vi "mqttCmdBuildPayloadInternal.vi"(8 "error in (no error)":errorcluster, 11 "mqttCmdConnect in":refnum<class "ConnectMqttMsg.lvclass">) -> (0 "error out":errorcluster, 2 "payload":u8[](array[numeric]) format="%x", 3 "mqttCmdConnect out":refnum<class "ConnectMqttMsg.lvclass">)   [LabVIEW 2020, in "ConnectMqttMsg.lvclass"]
uses:
  ConnectMqttMsg.lvclass
  ConnectMqttMsg.lvclass/ConnectMqttMsg.ctl
  BaseMqttMsg.lvclass
panel:
  out "willMessage out":u8[](array[numeric])
  out "userInfo out":u8[](array[numeric])
  out "clientID out":u8[](array[numeric])
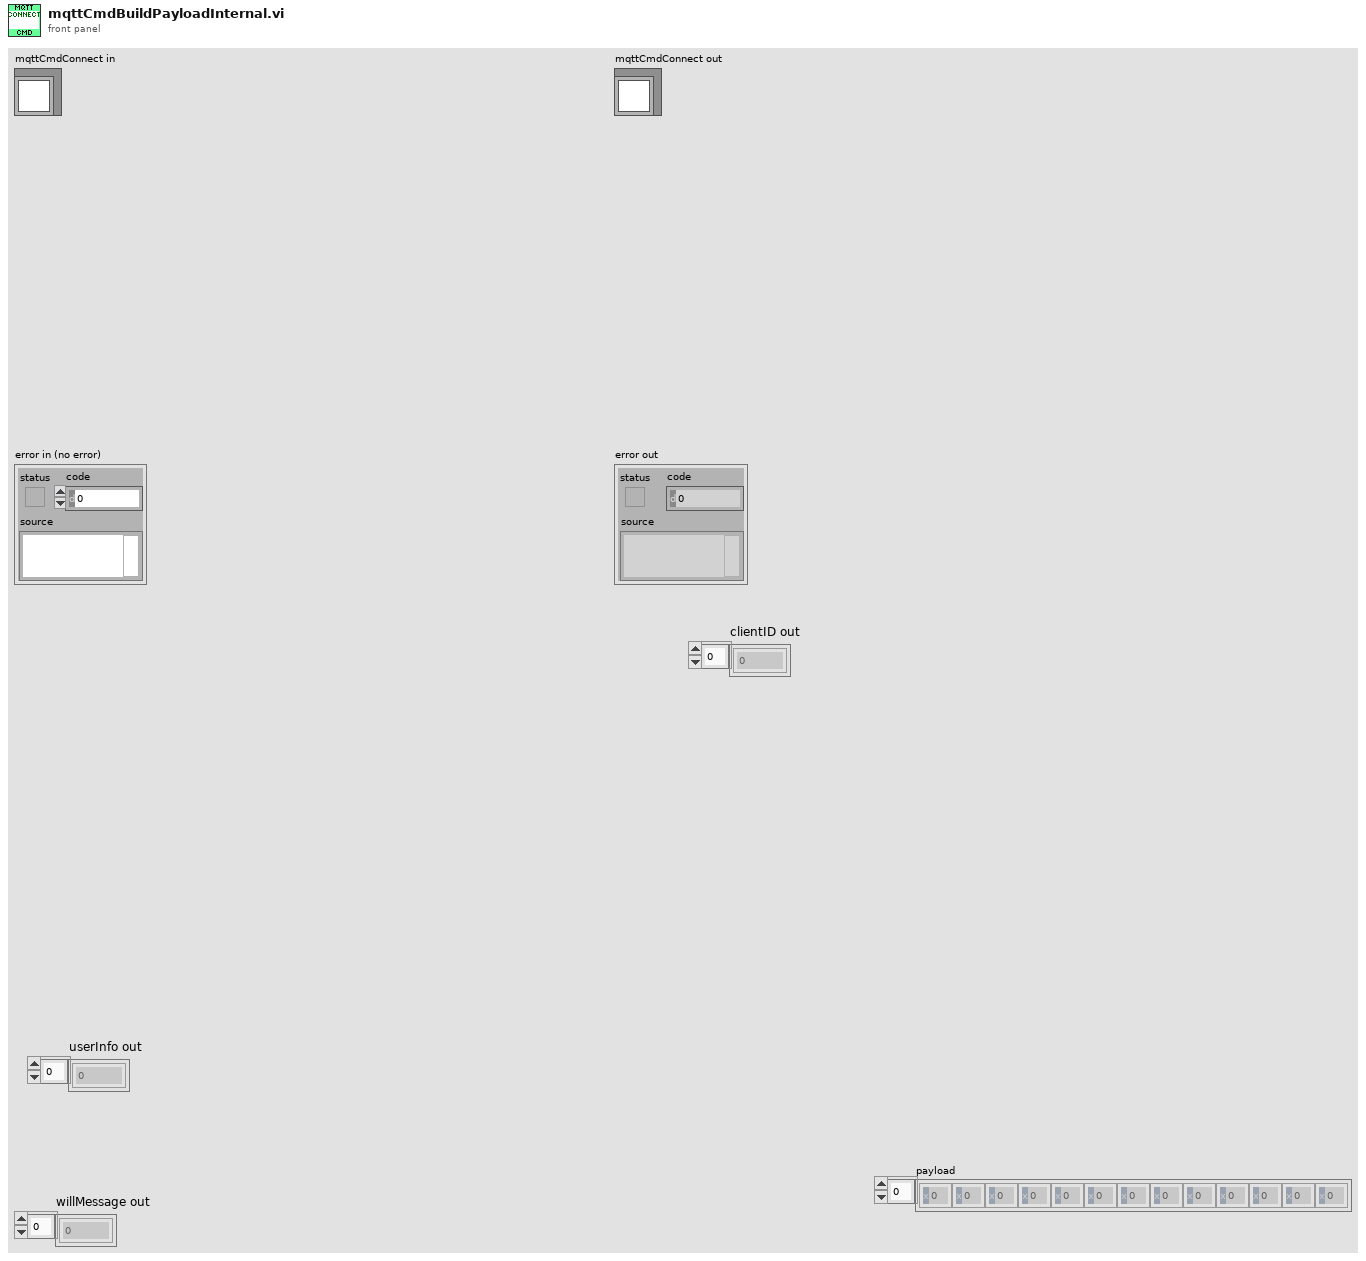
[diagram p1: front panel]
types:
  T1 = typedef "MQTT Client.lvclass/WillDefinition.ctl" = cluster{"Will message":string, "Will Topic":string}
  T2 = typedef "MQTT Client.lvclass/UserCredentials.ctl" = cluster{"User Name":string, "Password":string}
  T3 = typedef "MQTT Client.lvclass/ConnectionFlags.ctl" = cluster{"user name":bool, "password":bool, "will retain":bool, "will flag":bool, "clean session":bool, "reserved":bool, "willQOS":enum8{"At most once", "At least once", "Exactly once", "Reserved"}}
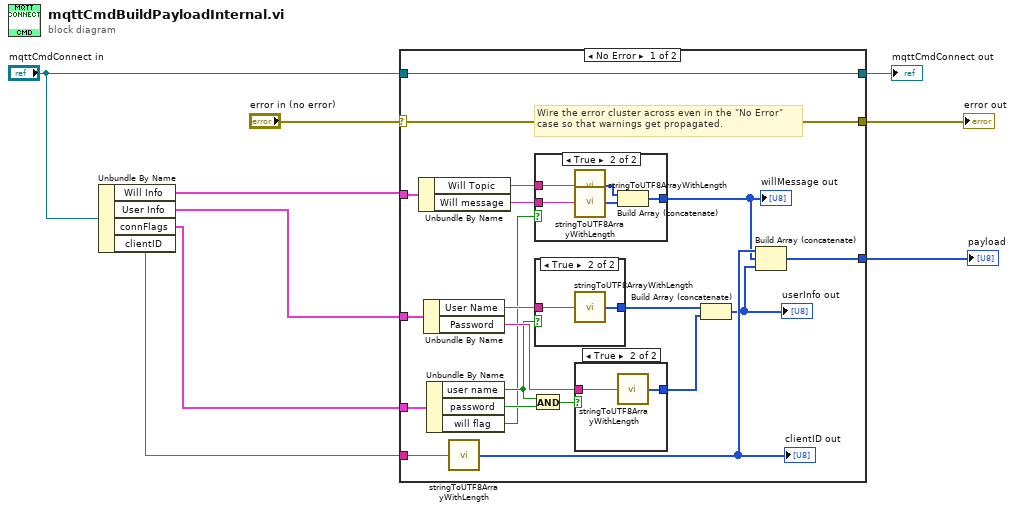
[diagram p0: block diagram]
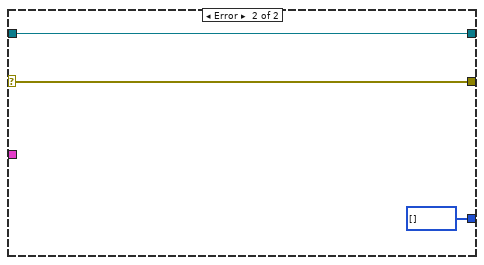
[diagram p5: hidden frame]
diagram:
  n1 = Unbundle By Name("mqttCmdConnect in") -> ("Will Info"=w4:T1, "User Info"=w3:T2, "connFlags"=w2:T3, "clientID"=w1:string)
  n2 = case shown="No Error" "error in (no error)" {
    selector: "error in (no error)" -> [w28 w41]
    tunnel: [w28 w41] -> w8
    tunnel: [w29 w40] -> w7
    tunnel: "mqttCmdConnect in" -> [w29 w40]
    tunnel: w1 -> [w27 _]
    tunnel: w2 -> [w19 _]
    tunnel: w3 -> [w16 _]
    tunnel: w4 -> [w11 _]
    tunnel: [w10 u8[] []] -> w6
    frame No Error {
      # "Wire the error cluster across even in the \"No Error\"\ncase so that warnings get propagated."
      n3 = Unbundle By Name(w11) -> ("Will Topic"=w14:string, "Will message"=w15:string)
      n4 = Unbundle By Name(w16) -> ("User Name"=w24:string, "Password"=w25:string)
      n5 = Unbundle By Name(w19) -> ("user name"=w18:bool, "password"=w17:bool, "will flag"=w12:bool)
      n6 = call "stringToUTF8ArrayWithLength.vi"("string"=w27) -> ("UTF8[]"=w26:u8[])  [unwired: 14 in]
      "clientID out" <- w26
      n7 = And(x=w18, y=w17) -> (x .and. y?=w21:bool)
      n8 = case shown="True" w12 {
        tunnel: w15 -> [_ w34]
        tunnel: w14 -> [_ w33]
        tunnel: [_ w30] -> w13
        frame False {
        }
        frame True {
          n9 = call "stringToUTF8ArrayWithLength.vi"("string"=w33) -> ("UTF8[]"=w32:u8[])  [unwired: 14 in]
          n10 = call "stringToUTF8ArrayWithLength.vi"("string"=w34) -> ("UTF8[]"=w31:u8[])  [unwired: 14 in]
          n11 = Build Array (concatenate)(w32, w31) -> (w30:u8[])
        }
      }
      "willMessage out" <- w13
      n12 = case shown="True" w18 {
        tunnel: w24 -> [_ w36]
        tunnel: [_ w35] -> w23
        frame False {
        }
        frame True {
          n13 = call "stringToUTF8ArrayWithLength.vi"("string"=w36) -> ("UTF8[]"=w35:u8[])  [unwired: 14 in]
        }
      }
      n14 = case shown="True" w21 {
        tunnel: w25 -> [_ w38]
        tunnel: [_ w37] -> w22
        frame False {
        }
        frame True {
          n15 = call "stringToUTF8ArrayWithLength.vi"("string"=w38) -> ("UTF8[]"=w37:u8[])  [unwired: 14 in]
        }
      }
      n16 = Build Array (concatenate)(w23, w22) -> (w20:u8[])
      "userInfo out" <- w20
      n17 = Build Array (concatenate)(w26, w13, w20) -> (w10:u8[])
    }
    frame Error {
    }
  }
  "error out" <- w8
  "mqttCmdConnect out" <- w7
  "payload" <- w6
